vi "lens forvard.vi"(9 "distance":dbl, 10 "focal":dbl, 11 "field":T1) -> (3 "field out":T1)   [LabVIEW 2012, in "Copy of LightPipes.lvlib"]
doc: "__declspec(dllexport) void lens_forvard (FIELD* field, double focal, double distance );"
uses:
  Copy of LightPipes.lvlib
  Debug/LightPipes.dll
panel:
  out "error out":errorcluster
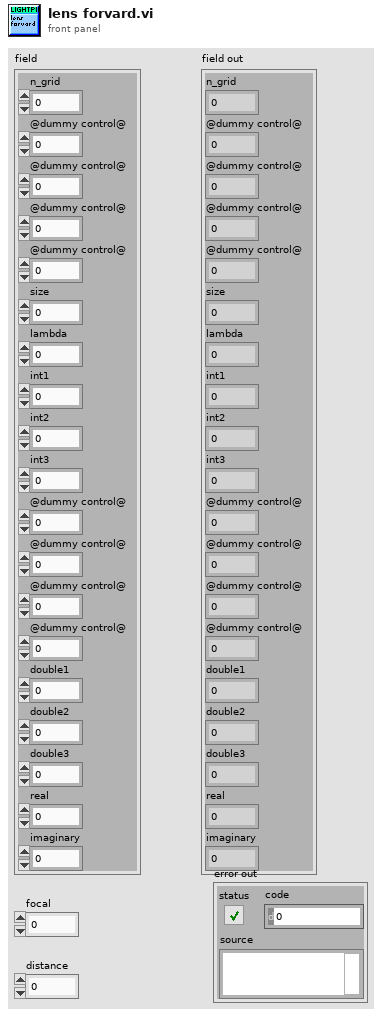
[diagram p1: front panel]
types:
  T1 = cluster{"n_grid":i32, "@dummy control@":i8, "@dummy control@":i8, "@dummy control@":i8, "@dummy control@":i8, "size":dbl, "lambda":dbl, "int1":i32, "int2":i32, "int3":i32, "@dummy control@":i8, "@dummy control@":i8, "@dummy control@":i8, "@dummy control@":i8, "double1":dbl, "double2":dbl, "double3":dbl, "real":u32, "imaginary":u32}
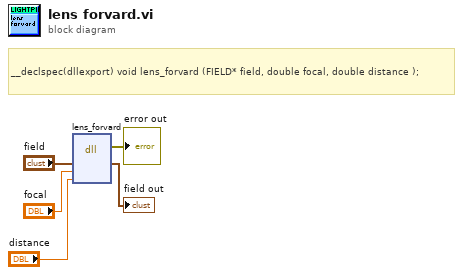
[diagram p0: block diagram]
diagram:
  # "__declspec(dllexport) void lens_forvard (FIELD* field, double focal, double distance );"
  n1 = dll-call lib="C:/Users/Green Beret/Documents/Visual Studio 2012/Projects/LightPipes/Debug/LightPipes.*" fn="lens_forvard"("field"="field", "focal_length"="focal", "distance"="distance") -> (error out=→"error out":errorcluster, "field"=→"field out":T1)  [unwired: 6 in, 1 out]
